vi "DAQ Engine.vi"(0 "DAQ Action":T1, 5 "LEDs":bool[](array[boolean]), 11 "Error In":errorcluster) -> (4 "Reset":bool, 6 "Keys":T2 caption="Keys inputs", 15 "Error Out":errorcluster)   [LabVIEW 2023]
doc: "VI for realizing DAQ action engine"
uses:
  Controls/Keys.ctl
  Controls/DAQ Actions.ctl
  <vilib>/DAQmx/read.llb/DAQmx Read (Digital 1D Bool 1Chan 1Samp).vi
  <vilib>/DAQmx/read.llb/DAQmx Read (Digital Bool 1Line 1Point).vi
  <vilib>/DAQmx/write.llb/DAQmx Write (Digital 1D Bool 1Chan 1Samp).vi
  <vilib>/DAQmx/create/channels.llb/DAQmx Create Channel (DI-Digital Input).vi
  <vilib>/DAQmx/create/channels.llb/DAQmx Create Channel (DO-Digital Output).vi
  <vilib>/DAQmx/miscellaneous.llb/DAQmx Fill In Error Info.vi
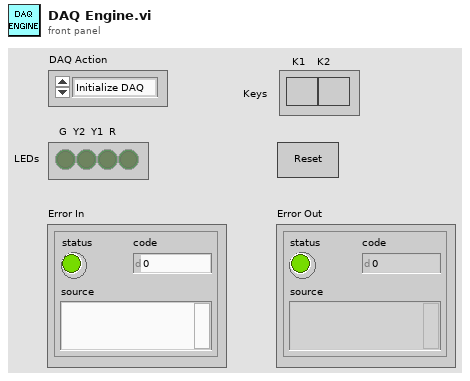
[diagram p1: front panel]
types:
  T1 = typedef "DAQ Actions.ctl" = enum16{"Initialize DAQ", "Read Keys", "Read Reset ", "Write LEDs", "Release DAQ"}
  T2 = typedef "Keys.ctl" = bool[]
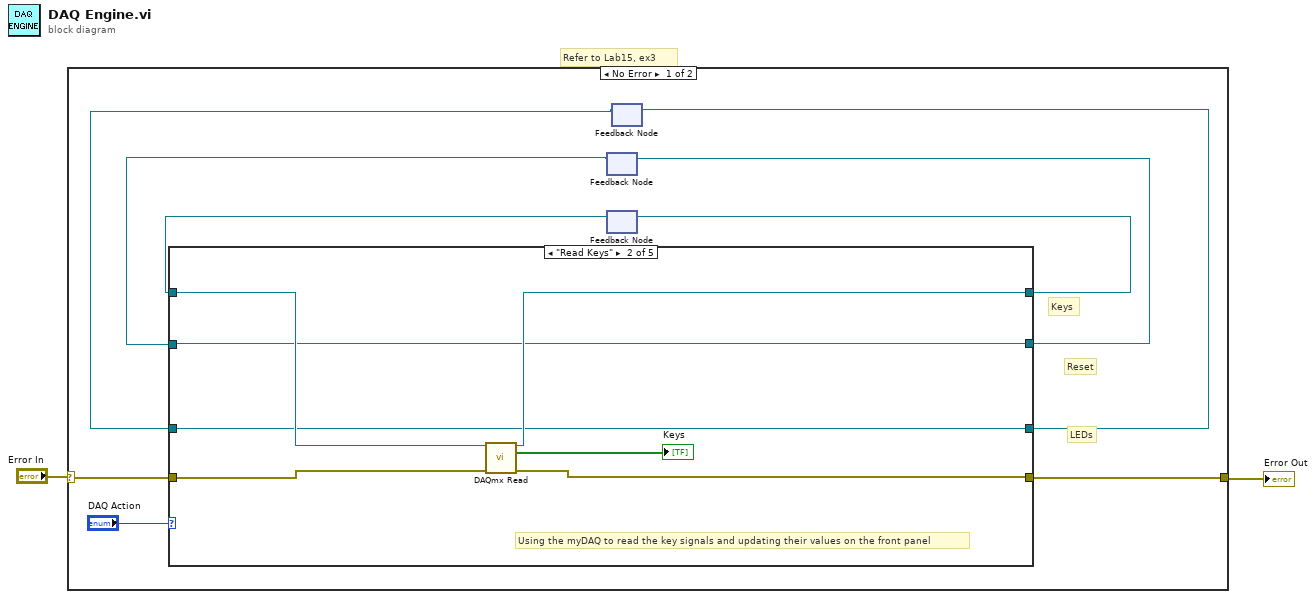
[diagram p0: block diagram]
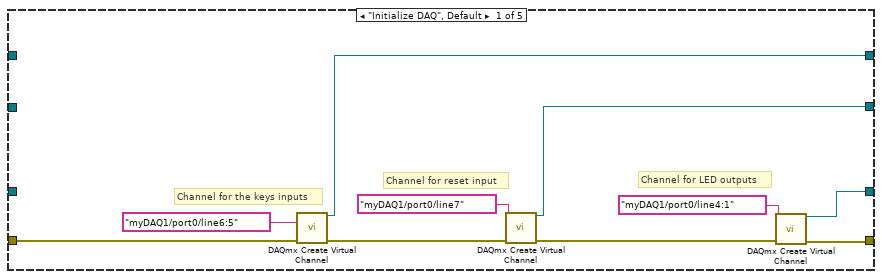
[diagram p2: hidden frame]
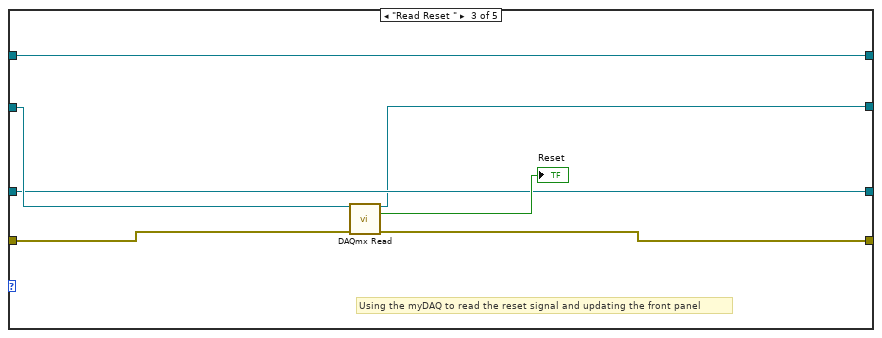
[diagram p3: hidden frame]
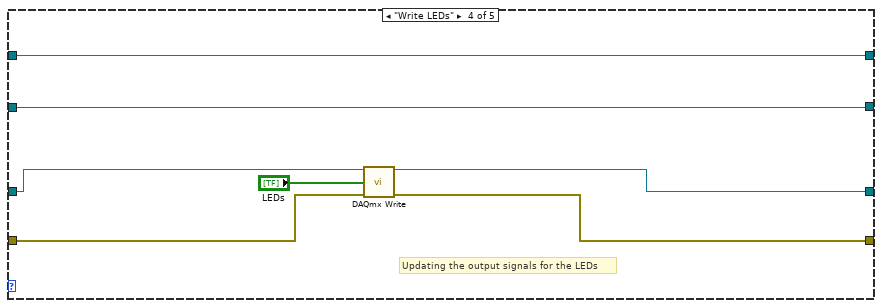
[diagram p4: hidden frame]
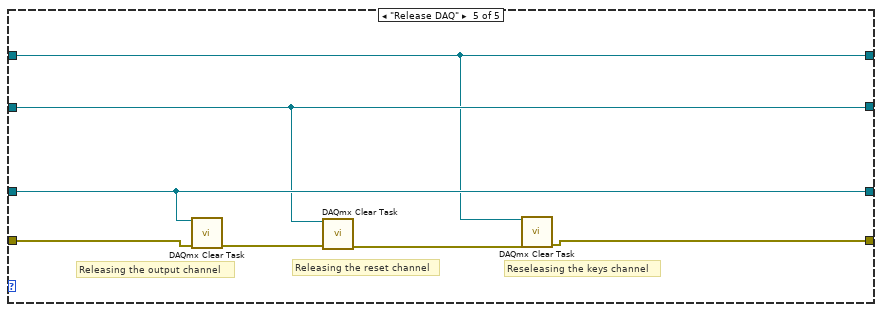
[diagram p5: hidden frame]
diagram:
  # "Refer to Lab15, ex3"
  n1 = case shown="No Error" "Error In" {
    selector: "Error In" -> [w10 w50]
    tunnel: [w9 w50] -> w1
    frame No Error {
      # "LEDs"
      # "Reset"
      # "Keys"
      n2 = feedback #1() -> (w5:refnum<k21>)  [unwired: 1 in]
      n3 = feedback #2() -> (w11:refnum<k21>)  [unwired: 1 in]
      n4 = feedback #3() -> (w3:refnum<k21>)  [unwired: 1 in]
      n5 = case shown="\"Read Keys\"" "DAQ Action" {
        tunnel: w11 -> [_ w26 w33 w36 w43]
        tunnel: w10 -> [w20 w28 w35 w39 w49]
        tunnel: [w18 w27 w34 w38 w46] -> w9
        tunnel: [w17 w25 w33 w36 w43] -> w8
        tunnel: [w14 w23 w29 w37 w44] -> w6
        tunnel: w5 -> [_ w23 w32 w37 w44]
        tunnel: [w12 w22 w30 w40 w45] -> w4
        tunnel: w3 -> [_ w22 w30 w42 w45]
        frame "Initialize DAQ", Default {
          # "Channel for LED outputs"
          # "Channel for reset input"
          # "Channel for the keys inputs"
          n6 = call-poly <vilib>:"DAQmx Create Virtual Channel.vi"("lines"=tag "myDAQ1/port0/line6:5", "error in"=w20) -> ("task out"=w17:refnum<k21>, "error out"=w21:errorcluster)  [unwired: 12 in]
          n7 = call-poly <vilib>:"DAQmx Create Virtual Channel.vi"("lines"=tag "myDAQ1/port0/line7", "error in"=w21) -> ("task out"=w14:refnum<k21>, "error out"=w19:errorcluster)  [unwired: 12 in]
          n8 = call-poly <vilib>:"DAQmx Create Virtual Channel.vi"("lines"=tag "myDAQ1/port0/line4:1", "error in"=w19) -> ("task out"=w12:refnum<k21>, "error out"=w18:errorcluster)  [unwired: 12 in]
        }
        frame "Read Keys" {
          # "Using the myDAQ to read the key signals and updating their values on the front panel"
          n9 = call-poly <vilib>:"DAQmx Read.vi"("task/channels in"=w26, "error in"=w28) -> ("task out"=w25:refnum<k21>, "data"=→"Keys":bool[], "error out"=w27:errorcluster)  [unwired: 11 in]
        }
        frame "Read Reset " {
          # "Using the myDAQ to read the reset signal and updating the front panel"
          n10 = call-poly <vilib>:"DAQmx Read.vi"("task/channels in"=w32, "error in"=w35) -> ("task out"=w29:refnum<k21>, "data"=→"Reset":bool, "error out"=w34:errorcluster)  [unwired: 11 in]
        }
        frame "Write LEDs" {
          # "Updating the output signals for the LEDs"
          n11 = call-poly <vilib>:"DAQmx Write.vi"("task/channels in"=w42, "data"="LEDs", "error in"=w39) -> ("task out"=w40:refnum<k21>, "error out"=w38:errorcluster)  [unwired: 10 in, 1 out]
        }
        frame "Release DAQ" {
          # "Reseleasing the keys channel"
          # "Releasing the reset channel"
          # "Releasing the output channel"
          n12 = call <vilib>:"DAQmx Clear Task.vi"("task in"=w45, "error in"=w49) -> ("error out"=w48:errorcluster)  [unwired: 13 in]
          n13 = call <vilib>:"DAQmx Clear Task.vi"("task in"=w44, "error in"=w48) -> ("error out"=w47:errorcluster)  [unwired: 13 in]
          n14 = call <vilib>:"DAQmx Clear Task.vi"("task in"=w43, "error in"=w47) -> ("error out"=w46:errorcluster)  [unwired: 13 in]
        }
      }
      n15 = feedback-in #1(w6) -> ()
      n16 = feedback-in #2(w8) -> ()
      n17 = feedback-in #3(w4) -> ()
    }
    frame Error {
    }
  }
  "Error Out" <- w1
